vi "SubVI_HandleFileChanges.vi"(0 "File Refnum in":refnum<k34>, 1 "Independent?":bool, 3 "notifier in":refnum<notifier>, 5 "Global File Information":T1, 7 "Sava data tured on or off?":bool, 9 "Save Data TDMS":bool, 11 "error in (no error)":errorcluster, 12 "File Info Changed?":bool, 13 "VI name":string="Sensors_DAQ") -> (4 "File Refnum out":refnum<k34>, 6 "Global File Information out":T1, 15 "error out":errorcluster)   [LabVIEW 2018]
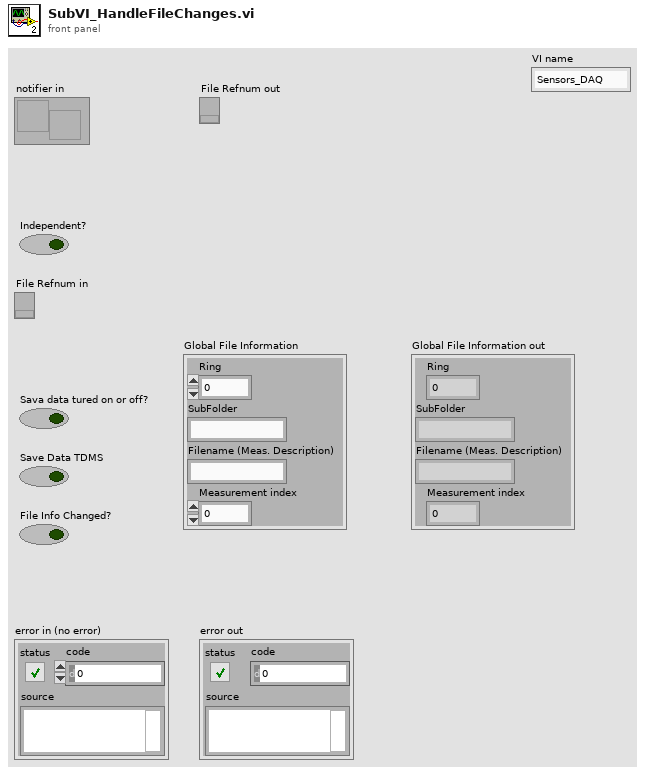
[diagram p1: front panel]
types:
  T1 = cluster{"Ring":u16, "SubFolder":string, "Filename (Meas. Description)":string, "Measurement index":i32}
  T2 = enum16{"open", "open or create", "create or replace", "create", "open (read-only)"}
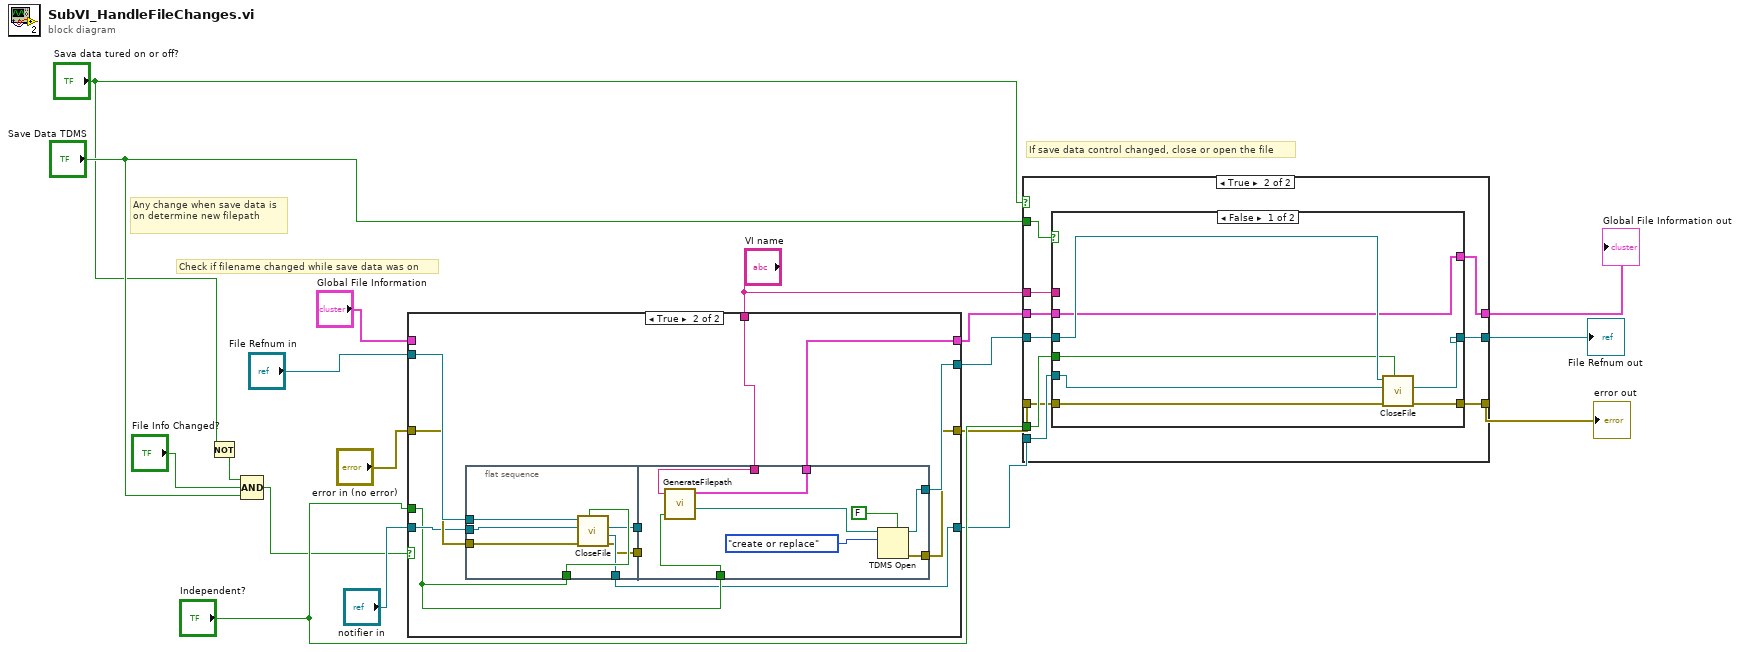
[diagram p0: block diagram]
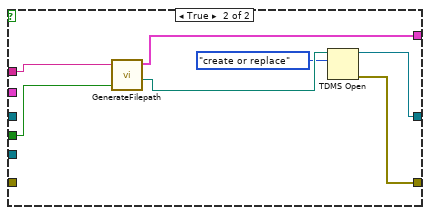
[diagram p4: hidden frame]
diagram:
  # "If save data control changed, close or open the file"
  # "Any change when save data is on determine new filepath"
  # "Check if filename changed while save data was on"
  n1 = Not(x="Sava data tured on or off?") -> (.not. x?=w5:bool)
  n2 = Compound Arithmetic op=AND(w5, "File Info Changed?", "Save Data TDMS") -> (w7:bool)
  n3 = case shown="True" w7 {
    tunnel: "notifier in" -> [w22 w28]
    tunnel: "Independent?" -> [_ w27]
    tunnel: [w22 w26] -> w11
    tunnel: "File Refnum in" -> [w20 w33]
    tunnel: "error in (no error)" -> [w21 w32]
    tunnel: [w20 w31] -> w16
    tunnel: [w21 w30] -> w17
    tunnel: "VI name" -> [_ w29]
    tunnel: "Global File Information" -> [w19 _]
    tunnel: [w19 w23] -> w2
    frame False {
    }
    frame True {
      n4 = flat-sequence {
        tunnel: w33 -> [w40]
        tunnel: w32 -> [w39]
        tunnel: w28 -> [w38]
        tunnel: w27 -> [w37]
        tunnel: [w36] -> w26
        tunnel: [w35] -> w25
        tunnel: [w34] -> w24
        tunnel: [w48] -> w31
        tunnel: [w47] -> w30
        tunnel: w29 -> [w46]
        tunnel: w27 -> [w45]
        tunnel: w25 -> [_]
        tunnel: w24 -> [_]
        tunnel: [w41] -> w23
        frame #0 {
          n5 = call "CloseFile.vi"("Independent?"=w37, "error in (no error)"=w39, "notifier in"=w38, "Refnum in"=w40) -> ("error out"=w34:errorcluster, "Notifier out"=w36:refnum<notifier>, "Not a refnum out"=w35:refnum<k34>)  [unwired: 4 in, 1 out]
        }
        frame #1 {
          n6 = call "GenerateFilepath.vi"("Instrument"=w46, "Check for file?"=w45) -> ("Global File Information"=w41:T1, "File Path Out"=w44:path)  [unwired: 3 in]
          n7 = TDMS Open(5:FALSE ("create index file? (T)"), 10:T2."create or replace" ("operation (0:open)"), 11:w44) -> (0:w47:errorcluster, 3:w48:refnum<k34>)  [unwired: 4 in]
        }
      }
    }
  }
  n8 = case shown="True" "Sava data tured on or off?" {
    tunnel: "Independent?" -> [_ w61]
    tunnel: w11 -> [_ w60]
    tunnel: [w51 w59] -> w14
    tunnel: [w50 w58] -> w15
    tunnel: w16 -> [w51 w57]
    tunnel: w17 -> [w50 w56]
    tunnel: "Save Data TDMS" -> [_ w55]
    tunnel: "VI name" -> [_ w54]
    tunnel: w2 -> [w49 w52]
    tunnel: [w49 w53] -> w1
    frame False {
    }
    frame True {
      n9 = case shown="False" w55 {
        tunnel: w61 -> [w64 w72]
        tunnel: w60 -> [w65 _]
        tunnel: w57 -> [w68 _]
        tunnel: w56 -> [w67 _]
        tunnel: [w63 w75] -> w59
        tunnel: [w66 w74] -> w58
        tunnel: w54 -> [_ w73]
        tunnel: [w62 w69] -> w53
        tunnel: w52 -> [w62 _]
        frame False {
          n10 = call "CloseFile.vi"("Independent?"=w64, "error in (no error)"=w67, "notifier in"=w65, "Refnum in"=w68) -> ("error out"=w66:errorcluster, "Not a refnum out"=w63:refnum<k34>)  [unwired: 4 in, 2 out]
        }
        frame True {
          n11 = call "GenerateFilepath.vi"("Instrument"=w73, "Check for file?"=w72) -> ("Global File Information"=w69:T1, "File Path Out"=w71:path)  [unwired: 3 in]
          n12 = TDMS Open(10:T2."create or replace" ("operation (0:open)"), 11:w71) -> (0:w74:errorcluster, 3:w75:refnum<k34>)  [unwired: 5 in]
        }
      }
    }
  }
  "error out" <- w15
  "File Refnum out" <- w14
  "Global File Information out" <- w1
